vi "savedwork.vi"() -> ()   [LabVIEW 2009]
uses:
  <vilib>/vision/NI_Vision_Development_Module.lvlib
panel:
  in  "Trigger action 2":u32(ring)=1 items=["Disabled", "Trigger start of acquisition", "Trigger start of each buffer list", "Trigger each buffer", "Trigger each line (linescan)", "Trigger end of acquisition"]
  in  "Trigger Type 2":u32(ring) items=["External", "RTSI", "ISO In"]
  in  "Live scan interface name":string="img0"
  out "Live saturation image 2":T1(plugin-control)
  out "Live image 2":T1(plugin-control)
  out "Histogram graph 2":T2(graph)
  in  "Live scan 2":bool
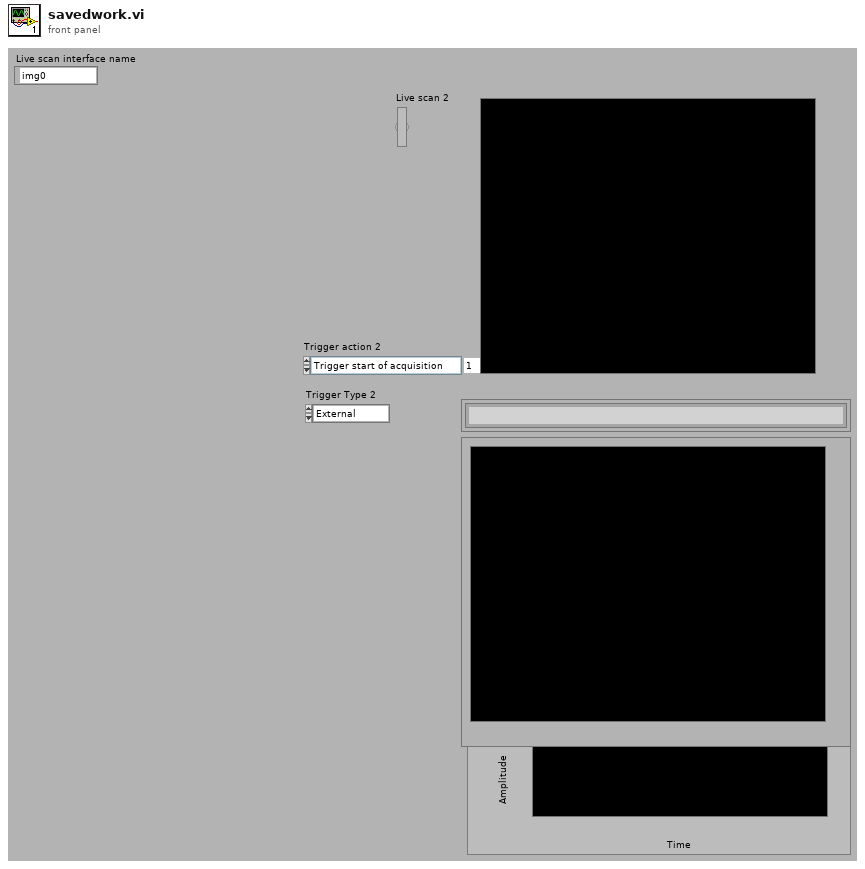
[diagram p1: front panel]
types:
  T1 = typedef "IMAQ Image.ctl" = refnum<image>
  T2 = cluster{"Starting Value":sgl, "Incremental Value":sgl, "Histogram":u32[]}
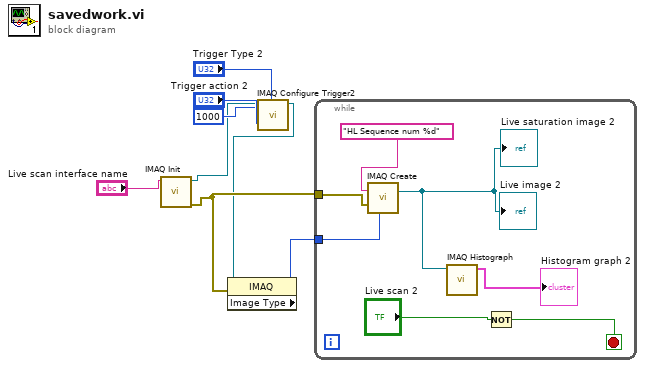
[diagram p0: block diagram]
diagram:
  n1 = call <vilib>:"IMAQ Init.vi"("Interface Name"="Live scan interface name") -> ("error out"=w7:errorcluster, "IMAQ Session Out"=w2:refnum<k11>)  [unwired: 9 in]
  n2 = call <vilib>:"IMAQ Configure Trigger2.vi"("Frame timeout (ms)"=u32 1000, "Trigger action"="Trigger action 2", "Trigger Type"="Trigger Type 2", "IMAQ Session In"=w2) -> ("IMAQ Session Out"=w1:refnum<k11>)  [unwired: 6 in, 1 out]
  n3 = property class="IMAQ"(reference=w1, error in=w7) -> ("Image Type"=w6:u32)  [unwired: 2 out]
  n4 = while {
    tunnel: w7 -> [w10]
    tunnel: w6 -> [w9]
    stop <- w12 stop-if-true
    n5 = call "IMAQ Create"("Image Name"="HL Sequence num %d" ("format string"), "Image Type"=w9, "error in (no error)"=w10) -> ("New Image"=w14:T1)  [unwired: 2 in, 1 out]
    "Live saturation image 2" <- w14
    "Live image 2" <- w14
    n6 = call "IMAQ Histograph"("Image"=w14) -> ("Histogram Graph"=→"Histogram graph 2":T2)  [unwired: 7 in, 3 out]
    n7 = Not(x="Live scan 2") -> (.not. x?=w12:bool)
  }
